vi "Import BrowerComponent.vi"(8 "error in (no error)":errorcluster, 9 "Parent Tag(\"\")":string, 10 "BrowerComponent in":refnum<class "BrowerComponent.lvclass">, 11 "BrowerController in":refnum<class "BrowerController.lvclass">) -> (0 "error out":errorcluster, 3 "BrowerController out":refnum<class "BrowerController.lvclass">)   [LabVIEW 2015, in "BrowerController.lvclass"]
uses:
  BrowerController.lvclass
  Models/BrowerComponent/BrowerComponent/BrowerComponent.lvclass
  BrowerController.lvclass/BrowerController.ctl
  Models/BrowerTree/Type Definition/Symbol Index.ctl
  Models/BrowerTree/BrowerTree.lvclass
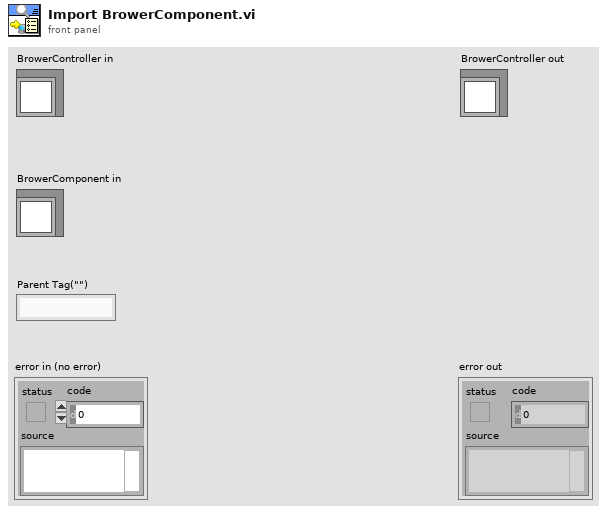
[diagram p1: front panel]
types:
  T1 = typedef "BrowerTree.lvclass/Symbol Index.ctl" = enum16{"PC", "Project", "Module", "DebugTask", "Communication"}
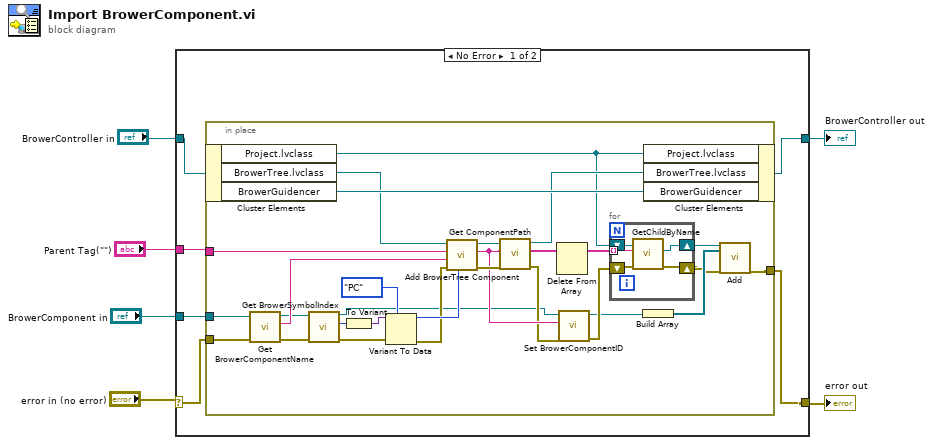
[diagram p0: block diagram]
diagram:
  n1 = case shown="No Error" "error in (no error)" {
    selector: "error in (no error)" -> [w12 w48]
    tunnel: [w11 w48] -> w5
    tunnel: [w9 w47] -> w3
    tunnel: "BrowerController in" -> [w10 w47]
    tunnel: "BrowerComponent in" -> [w8 _]
    tunnel: "Parent Tag(\"\")" -> [w7 _]
    frame No Error {
      n2 = in-place {
        in-place-border: w12 -> [w41]
        in-place-border: w7 -> [w40]
        in-place-border: [w36] -> w11
        in-place-border: w8 -> [w13]
        n3 = in-place-cluster #1(w10) -> ("Project.lvclass"=w35:refnum<class "BrowerComponent.lvclass">, "BrowerTree.lvclass"=w38:refnum<class "BrowerTree.lvclass">, "BrowerGuidencer"=w39:refnum<class "BrowerGuidencer.lvclass">)
        n4 = call "Get BrowerComponentName.vi"("error in (no error)"=w41, "BrowerComponent in"=w13) -> ("error out"=w21:errorcluster, "ComponentName"=w34:string, "BrowerComponent out"=w22:refnum<class "BrowerComponent.lvclass">)  [unwired: 7 in]
        n5 = call "Get BrowerSymbolIndex.vi"("error in (no error)"=w21, "BrowerComponent in"=w22) -> ("error out"=w19:errorcluster, "SymbolIndex"=w20:i32, "BrowerComponent out"=w14:refnum<class "BrowerComponent.lvclass">)  [unwired: 7 in]
        n6 = To Variant(anything=w20) -> (Variant=w18:variant)
        n7 = Variant To Data(error in=w19, type=Symbol_Index."PC" ("SymbolIndex"), Variant=w18) -> (data=w16:T1, error out=w15:errorcluster)
        n8 = call "Add BrowerTree Component.vi"("SymbolIndex"=w16, "error in (no error)"=w15, "Left Cell String"=w34, "Parent Tag"=w40, "BrowerTree in"=w38) -> ("error out"=w33:errorcluster, "BrowerComponentID(\"\")"=w31:string, "BrowerTree out"=w32:refnum<class "BrowerTree.lvclass">)  [unwired: 4 in]
        n9 = call "Get ComponentPath.vi"("error in (no error)"=w33, "BrowerComponentID(\"\")"=w31, "BrowerTree in"=w32) -> ("error out"=w30:errorcluster, "Navigate Tree:Get Paths"=w25:string[], "BrowerTree out"=w37:refnum<class "BrowerTree.lvclass">)  [unwired: 6 in]
        n10 = Delete From Array(array=w25) -> (array with subset deleted=w24:string[])  [unwired: 2 in, 1 out]
        n11 = call "Set BrowerComponentID.vi"("error in (no error)"=w30, "ComponentID(\"\")"=w31, "BrowerComponent in"=w14) -> ("error out"=w29:errorcluster, "BrowerComponent out"=w28:refnum<class "BrowerComponent.lvclass">)  [unwired: 7 in]
        n12 = for {
          tunnel: w24 -> [w45] mode=indexing
          shift-right: [w43] -> w23
          shift-left: w35 -> [w46]
          shift-right: [w42] -> w26
          shift-left: w29 -> [w44]
          n13 = call-dynamic "GetChildByName.vi"("error in (no error)"=w44, "BrowerComponentID(\"\")"=w45, "reference in"=w46) -> ("error out"=w42:errorcluster, "BrowerComponent"=w43:refnum<class "BrowerComponent.lvclass">)  [unwired: 6 in, 1 out]
        }
        n14 = Build Array(w28) -> (w27:refnum<class "BrowerComponent.lvclass">[])
        n15 = in-place-cluster #1("Project.lvclass"=w35, "BrowerTree.lvclass"=w37, "BrowerGuidencer"=w39) -> (w9:refnum<class "BrowerController.lvclass">)
        n16 = call-dynamic "Add.vi"("reference in"=w23, "BrowerComponents"=w27, "error in (no error)"=w26) -> ("error out"=w36:errorcluster)  [unwired: 15 in, 1 out]
      }
    }
    frame Error {
    }
  }
  "error out" <- w5
  "BrowerController out" <- w3
